vi "Berechnung.vi"(6 "Enum":enum16{"Lesen", "Berechnen"}(ring), 8 "s":bool, 9 "Komp Dry":sgl, 10 "H2O":sgl, 11 "Komp. Wet":sgl) -> (0 "Komp Dry":sgl, 1 "H2O Ist":sgl, 2 "Interference":sgl, 3 "Komp. Wet errechnet":sgl, 4 "Komp. Wet":sgl)   [LabVIEW 2020, in "EPA 1065.lvlib" / "HovaCAL Interference verificaton.lvlib"]
uses:
  HovaCAL Interference verificaton.lvlib
  Visualisierungs Elemente/Auswahlfeld.ctl
panel:
  in  "Gas-Auswahl":T1
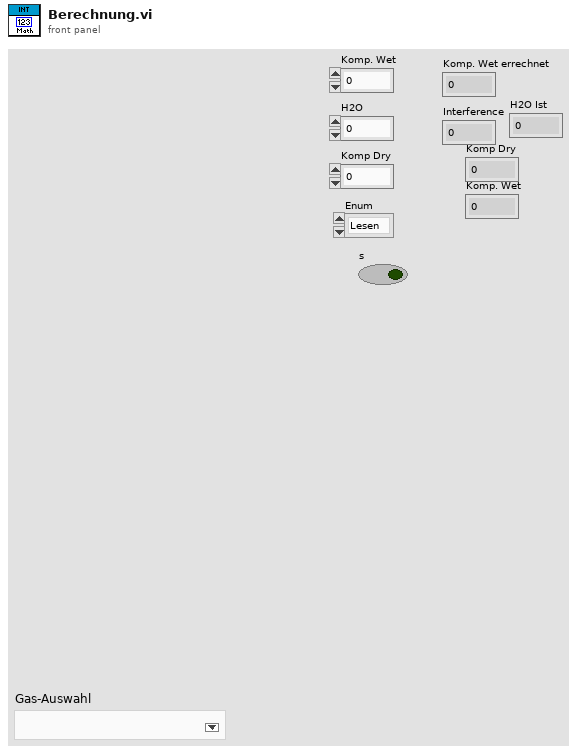
[diagram p1: front panel]
types:
  T1 = typedef "Auswahlfeld.ctl" = u16
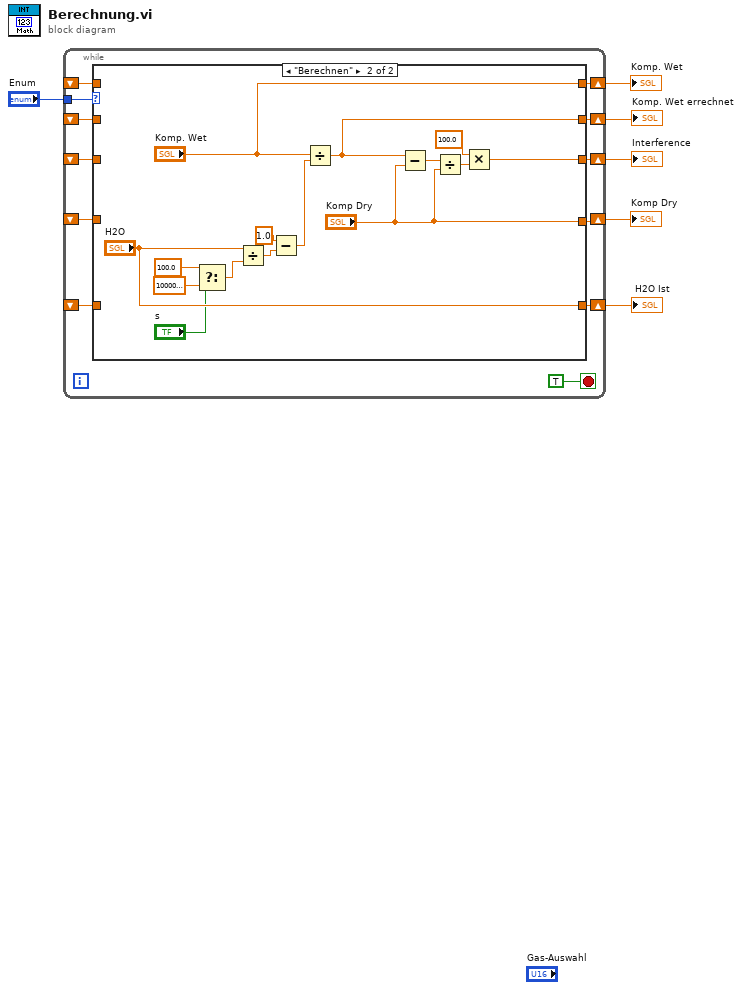
[diagram p0: block diagram]
diagram:
  n1 = while {
    shift-right: [w16] -> w5
    shift-left: _ -> [w9]
    shift-right: [w17] -> w6
    shift-left: _ -> [w10]
    shift-right: [w15] -> w4
    shift-left: _ -> [w7]
    shift-right: [w14] -> w3
    shift-left: _ -> [w8]
    shift-right: [w13] -> w2
    shift-left: _ -> [w11]
    tunnel: "Enum" -> [w12]
    stop <- TRUE stop-if-true
    n2 = case shown="\"Berechnen\"" w12 {
      tunnel: [w22 w34] -> w17
      tunnel: [w21 w33] -> w16
      tunnel: [w19 "H2O"] -> w15
      tunnel: [w20 "Komp Dry"] -> w14
      tunnel: [w23 "Komp. Wet"] -> w13
      tunnel: w11 -> [w23 _]
      tunnel: w10 -> [w22 _]
      tunnel: w9 -> [w21 _]
      tunnel: w8 -> [w20 _]
      tunnel: w7 -> [w19 _]
      frame "Lesen", Default {
      }
      frame "Berechnen" {
        n3 = Select(t=sgl 100.0, s="s", f=sgl 1000000.0 ("y")) -> (s? t:f=w24:sgl)
        n4 = Divide(x="H2O", y=w24) -> (x/y=w31:sgl)
        n5 = Subtract(x=sgl 1.0, y=w31) -> (x-y=w38:sgl)
        n6 = Divide(x="Komp. Wet", y=w38) -> (x/y=w34:sgl)
        n7 = Subtract(x=w34, y="Komp Dry") -> (x-y=w37:sgl)
        n8 = Divide(x=w37, y="Komp Dry") -> (x/y=w35:sgl)
        n9 = Multiply(x=sgl 100.0, y=w35) -> (x*y=w33:sgl)
      }
    }
  }
  "Komp. Wet errechnet" <- w6
  "Interference" <- w5
  "H2O Ist" <- w4
  "Komp Dry" <- w3
  "Komp. Wet" <- w2
